vi "SequenceGenerator (SubVI).vi"(11 "Array in":dbl[][](array[numeric])) -> (3 "Array":i8[](array[numeric]))   [LabVIEW 2014]
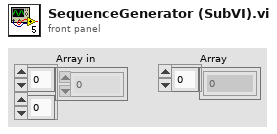
[diagram p1: front panel]
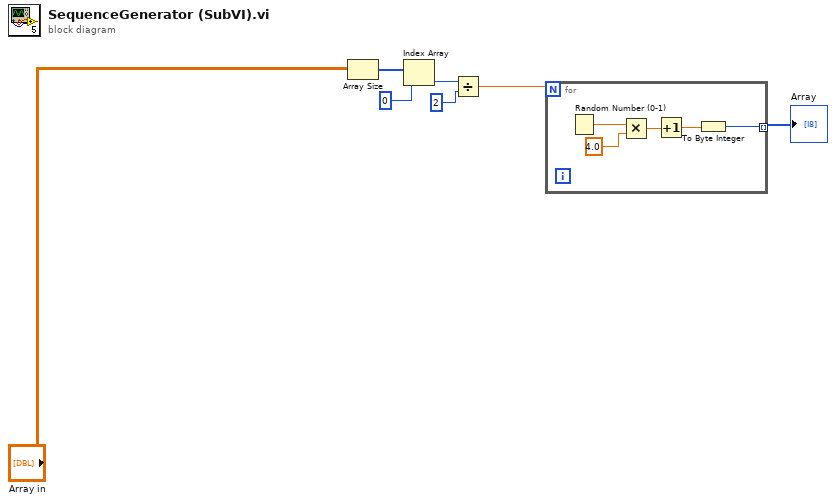
[diagram p0: block diagram]
diagram:
  n1 = Array Size(array="Array in") -> (size(s)=w7:i32[])
  n2 = Index Array(array=w7, index=0) -> (element=w1:i32)
  n3 = Divide(x=w1, y=2) -> (x/y=w2:dbl)
  n4 = for {
    N: w2 -> [_]
    tunnel: [w8] -> w5 mode=indexing
    n5 = Random Number (0-1)() -> (number: 0 to 1=w12:dbl)
    n6 = Multiply(x=w12, y=4.0) -> (x*y=w10:dbl)
    n7 = Increment(x=w10) -> (x+1=w9:dbl)
    n8 = To Byte Integer(number=w9) -> (8bit integer=w8:i8)
  }
  "Array" <- w5
